vi "IdentificaçãoHost.vi"() -> ()   [LabVIEW 2018]
uses:
  Tanque.ctl
  SMHostEnum.ctl
  <vilib>/addons/System Identification/Model Typedefs.llb/si_generic model.ctl
  <vilib>/addons/System Identification/Model Typedefs.llb/SI Model Type.ctl
  <vilib>/addons/System Identification/Model Typedefs.llb/si_variables.ctl
  Setpoints.ctl
  PRBSparameters.ctl
  <vilib>/addons/System Identification/NI_SysID.lvlib
panel:
  in  "Amplitude":dbl=0.5
  in  "Update setpoints":bool
  out "Output 2":dbl[][](graph)
  out "Estimated MIMO State-space Model":picture
  out "Output 1":dbl[][](graph)
  in  "Excitation duration":i32=120
  in  "Period":i32=20
  in  "Pump seed 2":i32
  in  "Pump seed 1":i32
  in  "Coletar":bool
  out "Tanks levels variation":cluster{dbl, dbl, dbl, dbl}(graph)
  out "Pump voltage variation":cluster{dbl, dbl}(graph)
  in  "Valvula proporcional 2":dbl=7.5
  in  "Valvula proporcional 1":dbl=7.5
  out "Tanque 4":T1 scale=0.0..20.0
  out "Tanque 3":T1 scale=0.0..20.0
  out "Tanque 2":T1 scale=0.0..20.0
  out "Tanque 1":T1 scale=0.0..20.0
  in  "Valvula 4":bool
  in  "Valvula 3":bool
  in  "Valvula 1":bool
  in  "Valvula 2":bool
  in  "Pump 2":dbl=3.0 min=0.0 format="%.2f"
  in  "Pump 1":dbl=3.0 min=0.0 format="%.2f"
  # "Sistema Tanque Quádruplo"
  # "PRBS excitation signal"
  # "[0-10V]"
  # "[0-10V]"
  # "[0-10V]"
  # "[0-10V]"
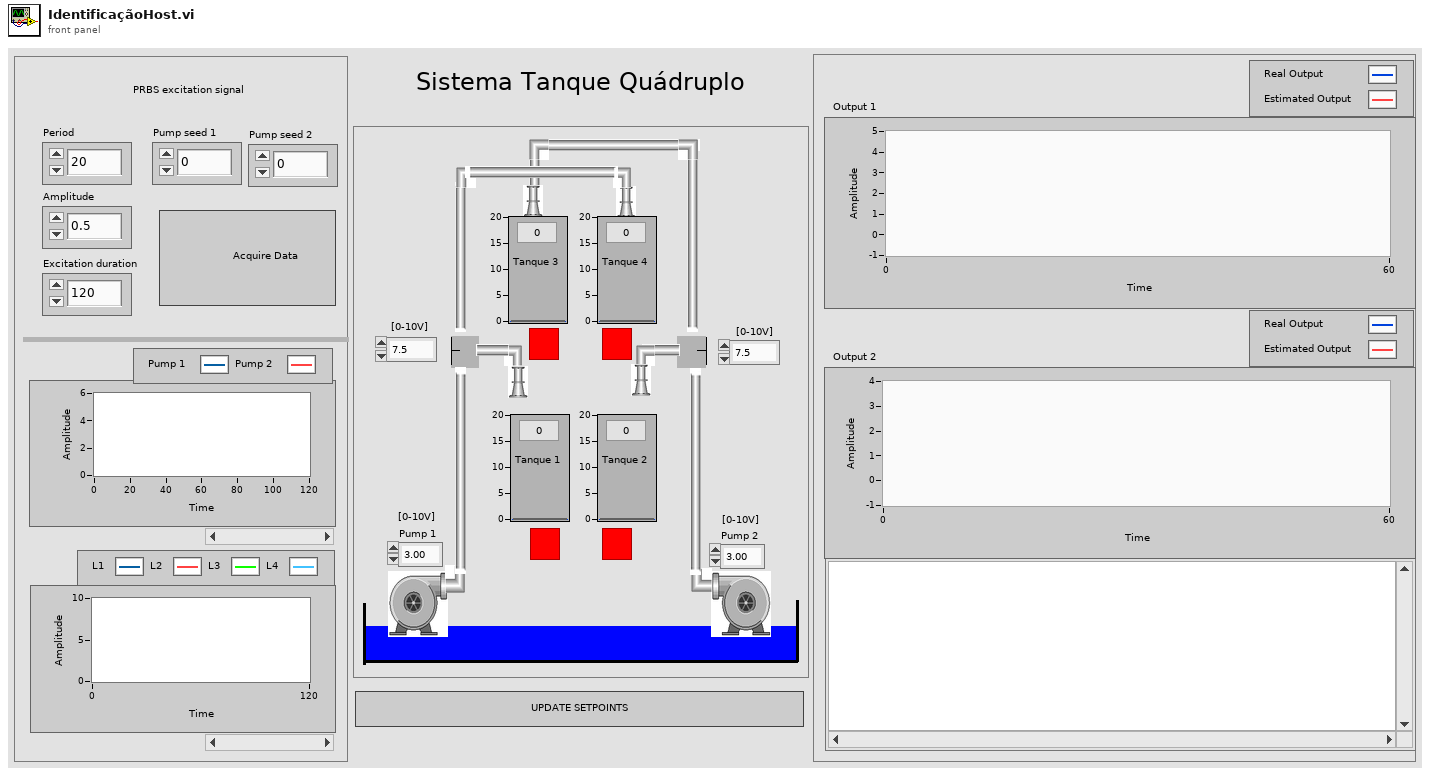
[diagram p1: front panel]
types:
  T1 = typedef "Tanque.ctl" = dbl
  T2 = typedef "SMHostEnum.ctl" = enum16{"Inicialização", "Pedir dados dos tanques", "Atualizar UI", "Configurar valores iniciais", "Começa aquisição", "Coletar dados", "Identificação", "Fecha arquivo log", "Data Logging", "Finalização"}
  T3 = typedef "Setpoints.ctl" = cluster{"Bomba 1":fxp<+/-,20,5>, "Bomba 2":fxp<+/-,20,5>, "Solenoide 1":bool, "Solenoide 2":bool, "Solenoide 3":bool, "Solenoide 4":bool, "Valvula proporcional 2":fxp<+/-,20,5>, "Valvula proporcional 1":fxp<+/-,20,5>}
  T4 = enum16{"open", "open or create", "create or replace", "create", "open (read-only)"}
  T5 = typedef "NI_SysID.lvlib/si_generic model.ctl" = cluster{"attributes":cluster{"version":string, "model type":T6, "input names":string[], "output names":string[], "notes":string}, "coefficients":cluster{"A ":dbl[][][], "B":dbl[][][], "F":dbl[][][], "C":dbl[][][], "D":dbl[][][]}, "std deviations":cluster{"A ":dbl[][][], "B":dbl[][][], "F":dbl[][][], "C":dbl[][][], "D":dbl[][][]}, "coefficients covariance":dbl[][][], "noise variance":dbl[][], "fs":dbl, "system info":cluster{"number of inputs":i32, "number of outputs":i32, "A order":i32[][], "B order":i32[][], "F order":i32[][], "C order":i32[][], "D order":i32[][], "Delays":i32[][]}, "kalman gain":dbl[][], "initial state":dbl[], "trans func":cluster{"betas":dbl[], "alphas":dbl[]}[][], "zeros-poles":cluster{"zeros":cdb[], "poles":cdb[], "gain":dbl}[][], "std of trans func":cluster{"betas":dbl[], "alphas":dbl[]}[][], "std of zeros-poles":cluster{"zeros":cdb[], "poles":cdb[], "gain":dbl}[][], "trans func (noise)":cluster{"betas":dbl[], "alphas":dbl[]}[][], "std of trans func (noise)":cluster{"betas":dbl[], "alphas":dbl[]}[][], "zeros-poles (noise)":cluster{"zeros":cdb[], "poles":cdb[], "gain":dbl}[][], "std of zeros-poles (noise)":cluster{"zeros":cdb[], "poles":cdb[], "gain":dbl}[][], "Symbolic State Space Model":cluster{"Symbolic A":string[][], "Symbolic B":string[][], "Symbolic C":string[][], "Symbolic D":string[][], "Symbolic K":string[][], "Symbolic Initial State":string[]}, "delay":dbl[][], "variables":T7, "grey trans func spec":cluster{"orders of TF model":cluster{" num order":i32, "den order":i32}, "# of zeros/poles at origin":cluster{"zeros/poles":u16, "number ":i32}, "delay initial?":bool, "gain initial?":bool}}
  T6 = typedef "NI_SysID.lvlib/SI Model Type.ctl" = u16
  T7 = typedef "NI_SysID.lvlib/si_variables.ctl" = cluster{"name":string, "initial guess":dbl, "upper limit":dbl, "lower limit":dbl, "value":dbl}[]
  T8 = enum8{"Enabled", "Disabled", "Disabled and Grayed Out"}
  T9 = typedef "PRBSparameters.ctl" = cluster{"seed":i64, "samples":i64, "upsampling factor":i32, "polynomial order":i32, "Amplitude":dbl}[]
  T10 = typedef "imagedata.ctl" = cluster{"image type":i32, "image depth":i32, "image":u8[], "mask":u8[], "colors":u32[], "Rectangle":cluster{"left":i16, "top":i16, "right":i16, "bottom":i16}}
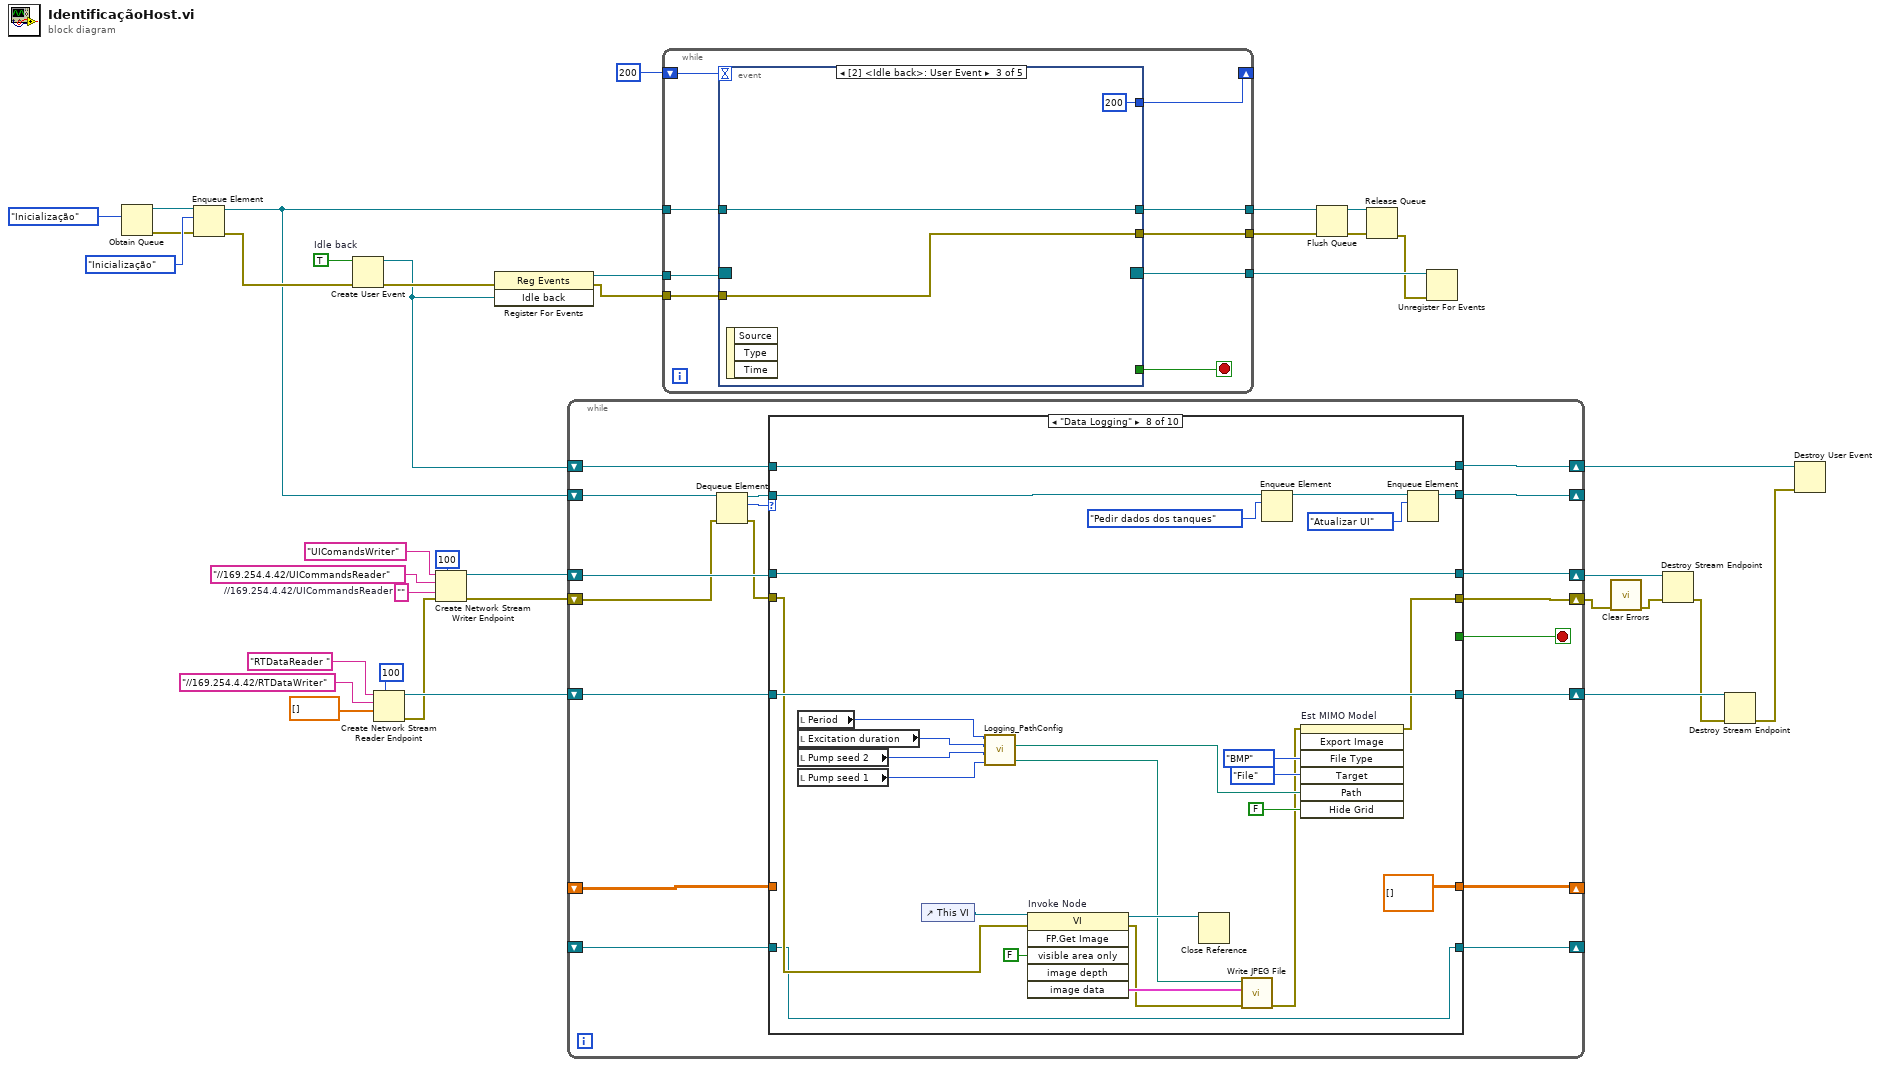
[diagram p0: block diagram]
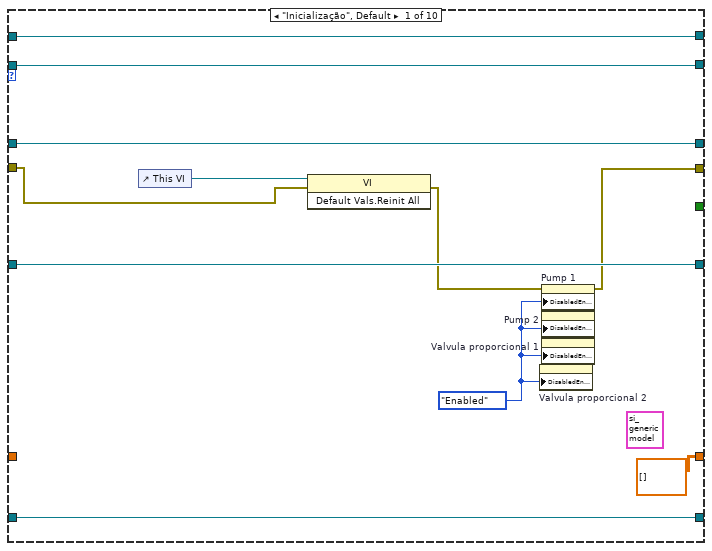
[diagram p2: hidden frame]
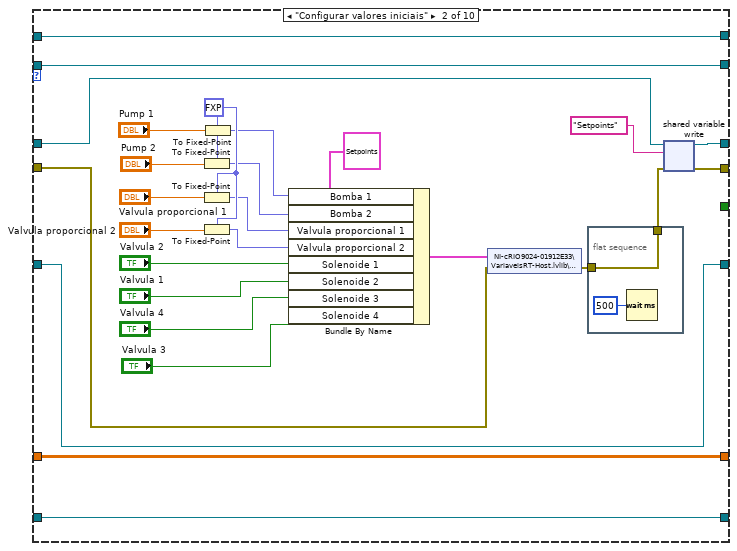
[diagram p3: hidden frame]
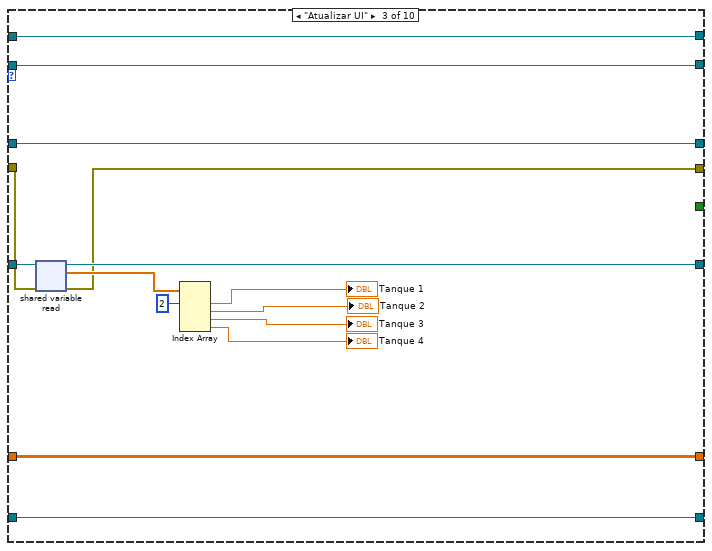
[diagram p4: hidden frame]
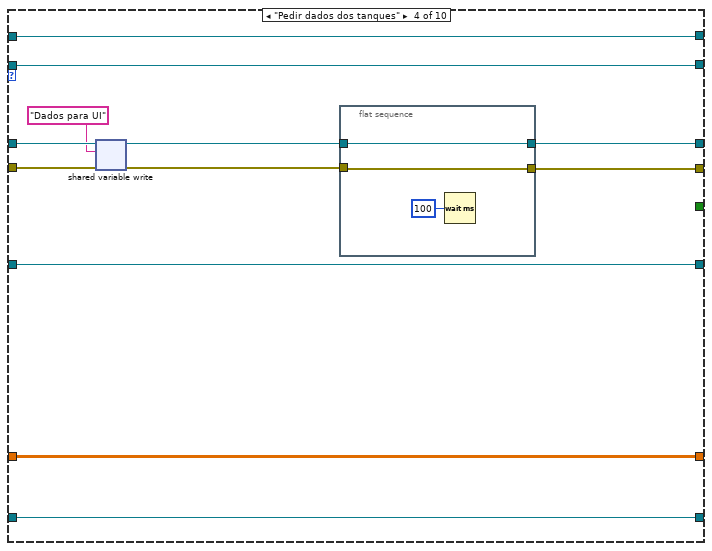
[diagram p5: hidden frame]
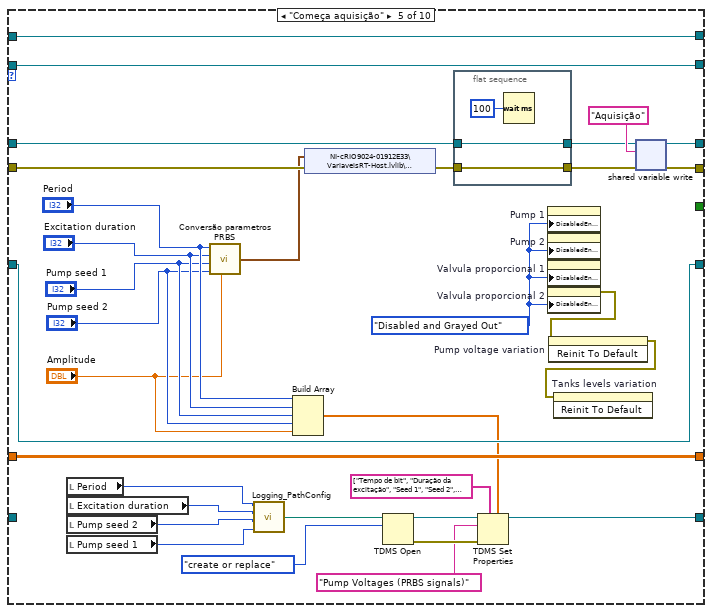
[diagram p6: hidden frame]
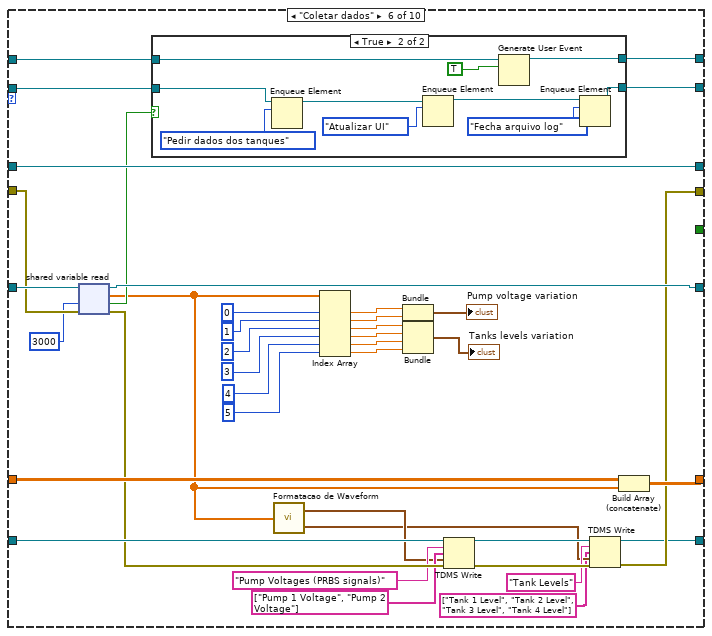
[diagram p7: hidden frame]
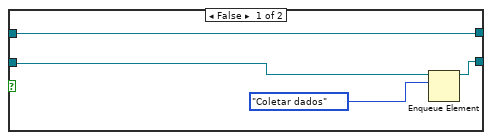
[diagram p8: hidden frame]
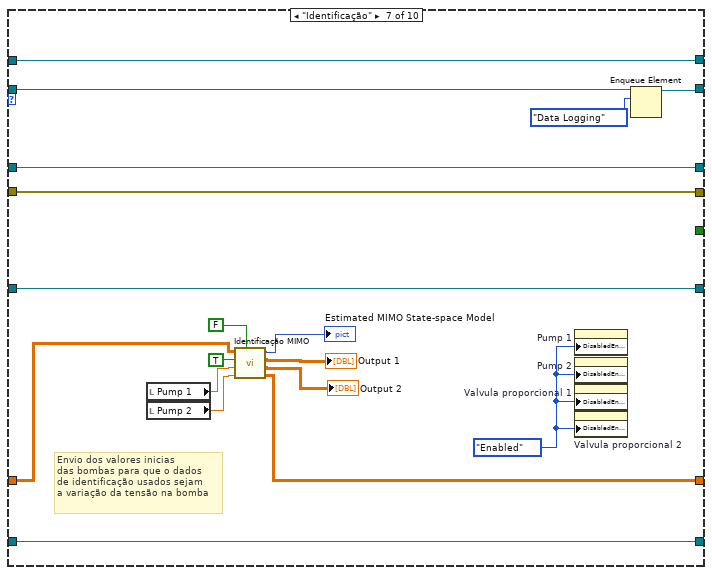
[diagram p9: hidden frame]
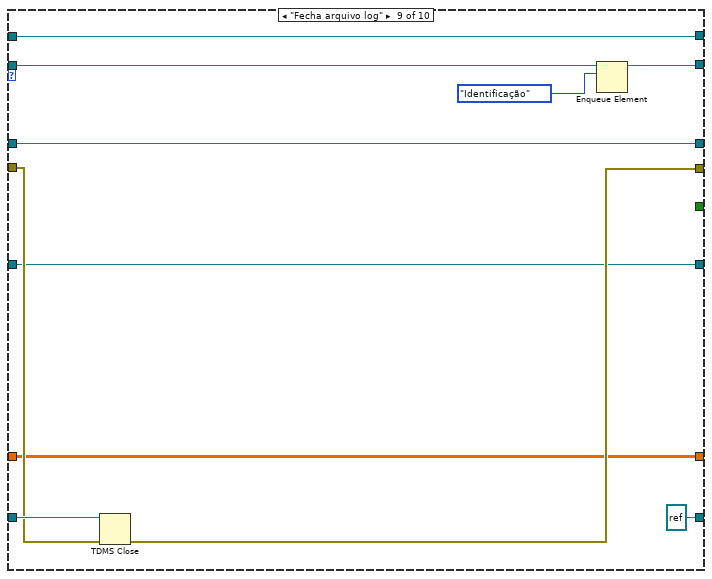
[diagram p10: hidden frame]
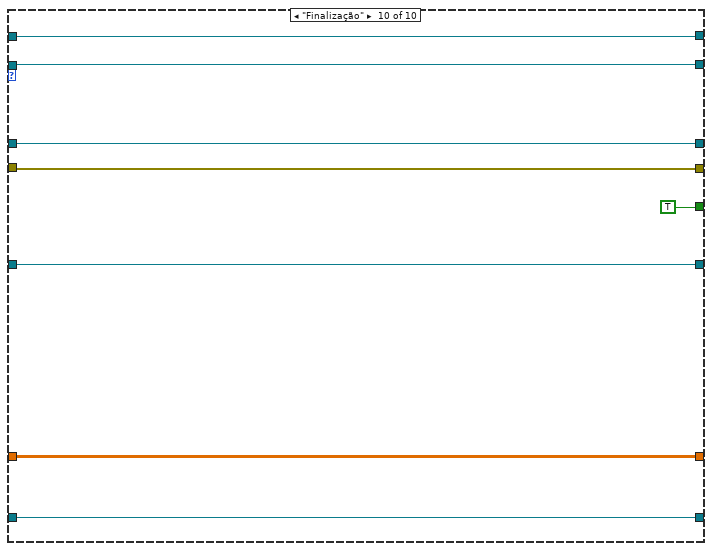
[diagram p11: hidden frame]
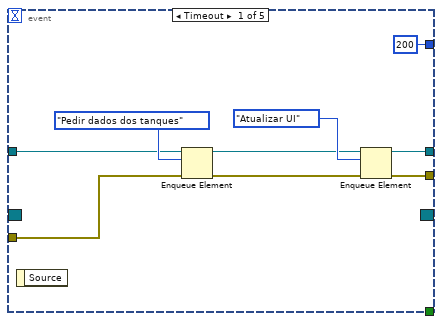
[diagram p12: hidden frame]
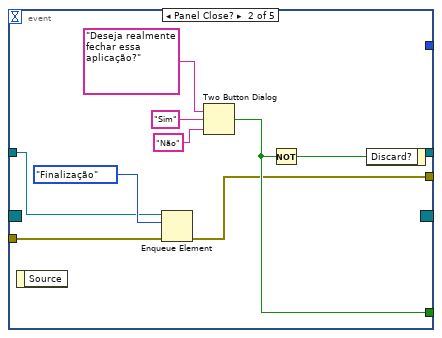
[diagram p13: hidden frame]
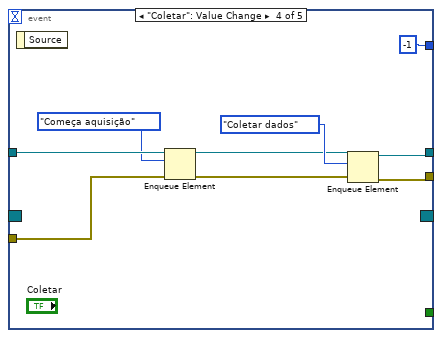
[diagram p14: hidden frame]
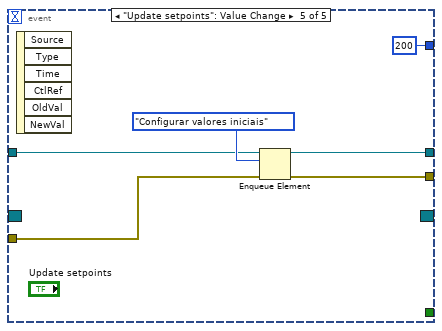
[diagram p15: hidden frame]
diagram:
  w19 = TRUE  # Idle back
  w26 = "//169.254.4.42/UICommandsReader"  # //169.254.4.42/UICommandsReader
  n1 = Obtain Queue(element data type=SMHostEnum."Inicialização") -> (queue out=w16:refnum<queue>, error out=w15:errorcluster)  [unwired: 4 in, 1 out]
  n2 = Enqueue Element(queue=w16, element=SMHostEnum."Inicialização", error in (no error)=w15) -> (queue out=w12:refnum<queue>, error out=w14:errorcluster)  [unwired: 1 in, 1 out]
  n3 = Create User Event(user event datatype=w19, error in=w14) -> (user event=w10:refnum<user-event>, error out=w17:errorcluster)
  n4 = Create Network Stream Reader Endpoint(7:100 ("reader buffer size"), 9:dbl[] [], 10:"//169.254.4.42/RTDataWriter" ("writer url"), 11:"RTDataReader " ("reader name")) -> (0:w23:errorcluster, 3:w33:refnum<k21>)  [unwired: 3 in]
  n5 = Create Network Stream Writer Endpoint(7:100 ("writer buffer size"), 8:w23, 9:"", 10:w26, 11:"UIComandsWriter") -> (0:w22:errorcluster, 3:w28:refnum<k21>)  [unwired: 2 in]
  n6 = register-events(error in=w17, w10) -> (reference out=w13:refnum<event-registration>, error out=w11:errorcluster)  [unwired: 1 in]
  n7 = while {
    shift-right: [w51] -> w6
    shift-left: w28 -> [w52]
    shift-right: [w39] -> w3
    shift-left: w22 -> [w45]
    shift-right: [w50] -> w5
    shift-left: w33 -> [w53]
    shift-right: [w48] -> _
    shift-left: w12 -> [w55]
    shift-right: [w47] -> _
    shift-left: _ -> [w46]
    shift-right: [w42] -> w7
    shift-left: w10 -> [w43]
    shift-right: [w41] -> _
    shift-left: _ -> [w40]
    stop <- w38 stop-if-true
    n8 = Dequeue Element(queue=w55, error in (no error)=w45) -> (queue out=w49:refnum<queue>, element=w54:T2, error out=w44:errorcluster)  [unwired: 1 in, 1 out]
    n9 = case shown="\"Data Logging\"" w54 {
      tunnel: w53 -> [w65 w75 w106 w119 w151 w200 w231 w255 w265 w275]
      tunnel: w44 -> [w60 w77 w100 w121 w157 w198 w230 w234 w269 w276]
      tunnel: w52 -> [w66 w80 w104 w122 w155 w199 w232 w254 w264 w277]
      tunnel: [w57 w78 w99 w115 w152 w169 w230 w235 w268 w276] -> w39
      tunnel: [w66 w76 w104 w116 w154 w199 w232 w254 w264 w277] -> w51
      tunnel: [w65 w75 w102 w119 w151 w194 w231 w255 w265 w275] -> w50
      tunnel: w49 -> [w64 w74 w101 w114 w150 w196 w227 w258 w261 w273]
      tunnel: [w64 w74 w101 w114 w150 w195 w228 w248 w260 w273] -> w48
      tunnel: [dbl[][] [] w71 w98 w113 w143 w179 w221 dbl[][] [] w266 w272] -> w47
      tunnel: w46 -> [_ w71 w98 w113 w143 w178 w216 _ w266 w272]
      tunnel: w43 -> [w62 w70 w97 w112 w149 w177 w226 w257 w263 w274]
      tunnel: [w62 w70 w97 w112 w149 w176 w226 w257 w263 w274] -> w42
      tunnel: [w56 w67 w96 w111 w127 w168 w215 w233 refnum<k34> refnum ("tdms file out") w271] -> w41
      tunnel: w40 -> [w56 w67 w96 w111 _ w174 w215 w233 w270 w271]
      tunnel: [_ _ _ _ _ _ _ _ _ TRUE] -> w38
      frame "Inicialização", Default {
        (unwired) T5 {"attributes"={"version"="v3.0", "model type"=0, "input names"=[], "output names"=[], "notes"=""}, "coefficients"={"A "=[], "B"=[], "F"=[], "C"=[], "D"=[]}, "std deviations"={"A "=[], "B"=[], "F"=[], "C"=[], "D"=[]}, "coefficients covariance"=[], "noise variance"=[], "fs"=0.0, "system info"={"number of inputs"=0, "number of outputs"=0, "A order"=[], "B order"=[], "F order"=[], "C order"=[], "D order"=[], "Delays"=[]}, "kalman gain"=[], "initial state"=[], "trans func"=[], "zeros-poles"=[], "std of trans func"=[], "std of zeros-poles"=[], "trans func (noise)"=[], "std of trans func (noise)"=[], "zeros-poles (noise)"=[], "std of zeros-poles (noise)"=[], "Symbolic State Space Model"={"Symbolic A"=[], "Symbolic B"=[], "Symbolic C"=[], "Symbolic D"=[], "Symbolic K"=[], "Symbolic Initial State"=[]}, "delay"=[], "variables"=[], "grey trans func spec"={"orders of TF model"={" num order"=1, "den order"=2}, "# of zeros/poles at origin"={"zeros/poles"=1, "number "=0}, "delay initial?"=FALSE, "gain initial?"=FALSE}} ("system model out")
        w59 = T8."Enabled" ("Disabled")
        n10 = control-ref of="This VI"() -> (w61:refnum<vi>)
        n11 = invoke class="VI" method="Default Vals.Reinit All"(reference=w61, error in=w60) -> (error out=w58:errorcluster)  [unwired: 1 in, 2 out]
        n12 = property on="Valvula proporcional 2" class="DigNum (strict)"("DisabledEnum"=w59) -> ()  [unwired: 2 in, 2 out]
        n13 = property on="Pump 1" class="DigNum (strict)"(error in=w58, "DisabledEnum"=w59) -> (error out=w57:errorcluster)  [unwired: 1 in, 1 out]
        n14 = property on="Pump 2" class="DigNum (strict)"("DisabledEnum"=w59) -> ()  [unwired: 2 in, 2 out]
        n15 = property on="Valvula proporcional 1" class="DigNum (strict)"("DisabledEnum"=w59) -> ()  [unwired: 2 in, 2 out]
      }
      frame "Configurar valores iniciais" {
        w91 = fxp<+/-,20,5> 0.0 ("fixed-point type")
        n16 = To Fixed-Point(fixed-point type=w91, number="Pump 2") -> (fixed-point=w88:fxp<+/-,20,5>)
        n17 = To Fixed-Point(fixed-point type=w91, number="Valvula proporcional 1") -> (fixed-point=w89:fxp<+/-,20,5>)
        n18 = To Fixed-Point(fixed-point type=w91, number="Valvula proporcional 2") -> (fixed-point=w90:fxp<+/-,20,5>)
        n19 = To Fixed-Point(fixed-point type=w91, number="Pump 1") -> (fixed-point=w87:fxp<+/-,20,5>)
        n20 = Bundle By Name(cluster=T3 {"Bomba 1"=0.0, "Bomba 2"=0.0, "Solenoide 1"=FALSE, "Solenoide 2"=FALSE, "Solenoide 3"=FALSE, "Solenoide 4"=FALSE, "Valvula proporcional 2"=0.0, "Valvula proporcional 1"=0.0} ("Cluster"), "Bomba 1"=w87, "Bomba 2"=w88, "Valvula proporcional 1"=w89, "Valvula proporcional 2"=w90, "Solenoide 1"="Valvula 2", "Solenoide 2"="Valvula 1", "Solenoide 3"="Valvula 4", "Solenoide 4"="Valvula 3") -> (w93:T3)
        n21 = shared-variable "NI-cRIO9024-01912E33\\VariaveisRT-Host.lvlib\\Setpoints"(w93, error in=w77) -> (error out=w73:errorcluster)
        n22 = flat-sequence {
          tunnel: w73 -> [w94]
          tunnel: [w94] -> w72
          frame #0 {
            n23 = Wait (ms)(milliseconds to wait=u32 500) -> ()  [unwired: 1 out]
          }
        }
        n24 = shared-variable-write(w80, w72, "Setpoints" ("data in")) -> (w76:refnum<k21>, w78:errorcluster)  [unwired: 1 in, 1 out]
      }
      frame "Atualizar UI" {
        n25 = shared-variable-read(w106, w100) -> (w102:refnum<k21>, w99:errorcluster, w103:dbl[])  [unwired: 1 in, 1 out]
        n26 = Index Array(array=w103, index #1=2 ("index")) -> (element #1=→"Tanque 1":dbl, element #2=→"Tanque 2":dbl, element #3=→"Tanque 3":dbl, element #4=→"Tanque 4":dbl)  [unwired: 3 in]
      }
      frame "Pedir dados dos tanques" {
        n27 = shared-variable-write(w122, w121, "Dados para UI" ("data in")) -> (w118:refnum<k21>, w117:errorcluster)  [unwired: 1 in, 1 out]
        n28 = flat-sequence {
          tunnel: w118 -> [w125]
          tunnel: w117 -> [w124]
          tunnel: [w125] -> w116
          tunnel: [w124] -> w115
          frame #0 {
            n29 = Wait (ms)(milliseconds to wait=u32 100) -> ()  [unwired: 1 out]
          }
        }
      }
      frame "Começa aquisição" {
        w148 = T8."Disabled and Grayed Out" ("Disabled")
        n30 = local read "Period"() -> (w142:i32)
        n31 = local read "Excitation duration"() -> (w141:i32)
        n32 = local read "Pump seed 2"() -> (w140:i32)
        n33 = local read "Pump seed 1"() -> (w139:i32)
        n34 = call "Conversão parametros PRBS.vi"("Amplitude"="Amplitude", "Seed bomba 2"="Pump seed 2", "Seed bomba 1"="Pump seed 1", "Duração da excitação (s)"="Excitation duration", "Periodo"="Period") -> ("PRBS Parameters 2"=w144:T9)  [unwired: 1 in]
        n35 = call "Logging_PathConfig.vi"("Period"=w142, "Excitation Duration"=w141, "Seed1"=w140, "Seed2"=w139) -> ("Data path 2"=w138:path)  [unwired: 1 in, 2 out]
        n36 = Build Array("Period", "Excitation duration", "Pump seed 1", "Pump seed 2", "Amplitude") -> (w130:dbl[])
        n37 = shared-variable "NI-cRIO9024-01912E33\\VariaveisRT-Host.lvlib\\PRBSparameters"(w144, error in=w157) -> (error out=w147:errorcluster)
        n38 = TDMS Open(10:T4."create or replace" ("operation (0:open)"), 11:w138) -> (0:w128:errorcluster, 3:w129:refnum<k34>)  [unwired: 5 in]
        n39 = flat-sequence {
          tunnel: w147 -> [w159]
          tunnel: [w160] -> w156
          tunnel: w155 -> [w160]
          tunnel: [w159] -> w153
          frame #0 {
            n40 = Wait (ms)(milliseconds to wait=u32 100) -> ()  [unwired: 1 out]
          }
        }
        n41 = TDMS Set Properties(5:w130, 7:string[] ["Tempo de bit", "Duração da excitação", "Seed 1", "Seed 2", "Amplitude"] ("property names"), 8:w128, 10:"Pump Voltages (PRBS signals)" ("group name"), 11:w129) -> (3:w127:refnum<k34>)  [unwired: 1 in, 3 out]
        n42 = property on="Pump 1" class="DigNum (strict)"("DisabledEnum"=w148) -> ()  [unwired: 2 in, 2 out]
        n43 = property on="Pump 2" class="DigNum (strict)"("DisabledEnum"=w148) -> ()  [unwired: 2 in, 2 out]
        n44 = property on="Valvula proporcional 1" class="DigNum (strict)"("DisabledEnum"=w148) -> ()  [unwired: 2 in, 2 out]
        n45 = property on="Valvula proporcional 2" class="DigNum (strict)"("DisabledEnum"=w148) -> (error out=w146:errorcluster)  [unwired: 2 in, 1 out]
        n46 = invoke on="Pump voltage variation" class="WFChart (strict)" method="Reinit To Default"(error in=w146) -> (error out=w145:errorcluster)  [unwired: 2 in, 2 out]
        n47 = invoke on="Tanks levels variation" class="WFChart (strict)" method="Reinit To Default"(error in=w145) -> ()  [unwired: 2 in, 3 out]
        n48 = shared-variable-write(w156, w153, "Aquisição" ("data in")) -> (w154:refnum<k21>, w152:errorcluster)  [unwired: 1 in, 1 out]
      }
      frame "Coletar dados" {
        n49 = shared-variable-read(w200, w198, 3000 ("timeout ms (-1)")) -> (w194:refnum<k21>, w173:errorcluster, w175:bool, w163:dbl[])
        n50 = case shown="True" w175 {
          tunnel: w196 -> [w203 w206]
          tunnel: [w202 w209] -> w195
          tunnel: w177 -> [w201 w213]
          tunnel: [w201 w211] -> w176
          frame False {
            n51 = Enqueue Element(queue=w203, element=SMHostEnum."Coletar dados") -> (queue out=w202:refnum<queue>)  [unwired: 2 in, 2 out]
          }
          frame True {
            n52 = Enqueue Element(queue=w206, element=SMHostEnum."Pedir dados dos tanques") -> (queue out=w207:refnum<queue>)  [unwired: 2 in, 2 out]
            n53 = Enqueue Element(queue=w207, element=SMHostEnum."Atualizar UI") -> (queue out=w210:refnum<queue>)  [unwired: 2 in, 2 out]
            n54 = Generate User Event(user event=w213, event data cluster=TRUE ("event data")) -> (user event out=w211:refnum<user-event>)  [unwired: 2 in, 1 out]
            n55 = Enqueue Element(queue=w210, element=SMHostEnum."Fecha arquivo log") -> (queue out=w209:refnum<queue>)  [unwired: 2 in, 2 out]
          }
        }
        n56 = call "Formatacao de Waveform.vi"("Array in"=w163) -> ("Tank Levels"=w164:waveform(dbl)[], "Pump Voltages"=w165:waveform(dbl)[])  [unwired: 2 in]
        n57 = Index Array(array=w163, index #1=0 ("index (row)"), index #2=1 ("index (row)"), index #3=2 ("index (row)"), index #4=3 ("index (row)"), index #5=4 ("index (row)"), index #6=5 ("index (row)")) -> (element #1=w187:dbl, element #2=w186:dbl, element #3=w185:dbl, element #4=w184:dbl, element #5=w182:dbl, element #6=w183:dbl)
        n58 = Bundle(w187, w186) -> (→"Pump voltage variation":cluster{dbl, dbl})  [unwired: 1 in]
        n59 = Bundle(w185, w184, w182, w183) -> (→"Tanks levels variation":cluster{dbl, dbl, dbl, dbl})  [unwired: 1 in]
        n60 = TDMS Write(0:w174, 5:"Pump Voltages (PRBS signals)" ("group name in (Untitled)"), 7:string[] ["Pump 1 Voltage", "Pump 2 Voltage"], 9:w165, 11:w173) -> (4:w171:refnum<k34>, 15:w170:errorcluster)  [unwired: 1 in, 2 out]
        n61 = TDMS Write(0:w171, 5:"Tank Levels" ("group name in (Untitled)"), 7:string[] ["Tank 1 Level", "Tank 2 Level", "Tank 3 Level", "Tank 4 Level"], 9:w164, 11:w170) -> (4:w168:refnum<k34>, 15:w169:errorcluster)  [unwired: 1 in, 2 out]
        n62 = Build Array (concatenate)(w178, w163) -> (w179:dbl[][])
      }
      frame "Identificação" {
        w225 = T8."Enabled" ("Disabled")
        # "Envio dos valores inicias\ndas bombas para que o dados \nde identificação usados sejam \na variação da tensão na bomba"
        n63 = local read "Pump 1"() -> (w219:dbl)
        n64 = local read "Pump 2"() -> (w220:dbl)
        n65 = call "Identificação MIMO.vi"("Remove Trend"=FALSE, "Init Pump 2 voltage"=w220, "Init Pump 1 voltage"=w219, "Invert indentification and validation data?"=TRUE, "Stimulus and Response Signal"=w216) -> ("Acquired and identification signals"=w221:dbl[][], "output 2"=→"Output 2":dbl[][], "output 1"=→"Output 1":dbl[][], "Estimated MIMO State-space Model"=→"Estimated MIMO State-space Model":picture)  [unwired: 2 in, 1 out]
        n66 = property on="Pump 1" class="DigNum (strict)"("DisabledEnum"=w225) -> ()  [unwired: 2 in, 2 out]
        n67 = property on="Pump 2" class="DigNum (strict)"("DisabledEnum"=w225) -> ()  [unwired: 2 in, 2 out]
        n68 = property on="Valvula proporcional 1" class="DigNum (strict)"("DisabledEnum"=w225) -> ()  [unwired: 2 in, 2 out]
        n69 = property on="Valvula proporcional 2" class="DigNum (strict)"("DisabledEnum"=w225) -> ()  [unwired: 2 in, 2 out]
        n70 = Enqueue Element(queue=w227, element=SMHostEnum."Data Logging") -> (queue out=w228:refnum<queue>)  [unwired: 2 in, 2 out]
      }
      frame "Data Logging" {
        n71 = local read "Period"() -> (w244:i32)
        n72 = local read "Excitation duration"() -> (w243:i32)
        n73 = local read "Pump seed 2"() -> (w242:i32)
        n74 = local read "Pump seed 1"() -> (w241:i32)
        n75 = control-ref of="This VI"() -> (w247:refnum<vi>)
        n76 = call "Logging_PathConfig.vi"("Period"=w244, "Excitation Duration"=w243, "Seed1"=w242, "Seed2"=w241) -> ("Model path"=w240:path, "Front panel image path"=w237:path)  [unwired: 1 in, 1 out]
        n77 = invoke on="Invoke Node" class="VI" method="FP.Get Image"(reference=w247, error in=w234, "visible area only"=FALSE ("Visible Area Only")) -> (reference out=w246:refnum<vi>, error out=w236:errorcluster, "image data"=w245:T10)  [unwired: 3 in, 3 out]
        n78 = Close Reference(reference=w246) -> ()  [unwired: 1 in, 1 out]
        n79 = call <vilib>:"Write JPEG File.vi"("error in (no error)"=w236, "image data"=w245, "path to JPEG file"=w237) -> ("error out"=w238:errorcluster)  [unwired: 7 in, 1 out]
        n80 = Enqueue Element(queue=w258, element=SMHostEnum."Pedir dados dos tanques") -> (queue out=w249:refnum<queue>)  [unwired: 2 in, 2 out]
        n81 = invoke on="Est MIMO Model" class="Pict" method="Export Image"(error in=w238, "File Type"=enum32{"BMP", "EPS", "EMF", "PICT"}."BMP", "Target"=enum32{"File", "Clipboard"}."File", "Path"=w240, "Hide Grid"=FALSE ("Always Overwrite")) -> (error out=w235:errorcluster)  [unwired: 2 in, 6 out]
        n82 = Enqueue Element(queue=w249, element=SMHostEnum."Atualizar UI") -> (queue out=w248:refnum<queue>)  [unwired: 2 in, 2 out]
      }
      frame "Fecha arquivo log" {
        n83 = TDMS Close(8:w269, 11:w270) -> (0:w268:errorcluster)  [unwired: 1 out]
        n84 = Enqueue Element(queue=w261, element=SMHostEnum."Identificação") -> (queue out=w260:refnum<queue>)  [unwired: 2 in, 2 out]
      }
      frame "Finalização" {
      }
    }
  }
  n85 = while {
    tunnel: w12 -> [w287]
    tunnel: [w286] -> w35
    tunnel: [w285] -> w34
    shift-right: [w283] -> _
    shift-left: 200 -> [w284]
    tunnel: w13 -> [w281]
    tunnel: w11 -> [w280]
    tunnel: [w279] -> w9
    stop <- w282 stop-if-true
    n86 = event shown="[2] <Idle back>: User Event" {
      selector: w281 -> [_ _ _ _ _]
      dyn-events: [_ _ _ _ _] -> w279
      timeout: w284 -> [_ _ _ _ _]
      tunnel: w287 -> [w295 w297 w308 w317 w322]
      tunnel: w280 -> [w294 w299 w307 w309 w321]
      tunnel: [w290 _ w308 w312 w320] -> w286
      tunnel: [w289 w298 w307 w310 w319] -> w285
      tunnel: [200 _ 200 -1 200] -> w283
      tunnel: [_ w301 _ _ _] -> w282
      event Timeout {
        n87 = event-data() -> ()  [unwired: 1 in, 1 out]
        n88 = Enqueue Element(queue=w295, element=SMHostEnum."Pedir dados dos tanques", error in (no error)=w294) -> (queue out=w291:refnum<queue>, error out=w288:errorcluster)  [unwired: 1 in, 1 out]
        n89 = Enqueue Element(queue=w291, element=SMHostEnum."Atualizar UI", error in (no error)=w288) -> (queue out=w290:refnum<queue>, error out=w289:errorcluster)  [unwired: 1 in, 1 out]
      }
      event Panel Close? {
        n90 = event-data() -> ()  [unwired: 1 in, 1 out]
        n91 = Enqueue Element(queue=w297, element=SMHostEnum."Finalização", error in (no error)=w299) -> (error out=w298:errorcluster)  [unwired: 1 in, 2 out]
        n92 = Two Button Dialog(message="Deseja realmente fechar essa aplicação?", 1:"Não" ("F button name (\"Cancel\")"), 2:"Sim" ("T button name (\"OK\")")) -> (T button?=w301:bool)
        n93 = Not(x=w301) -> (.not. x?=w302:bool)
        n94 = event-data("Discard?"=w302) -> ()  [unwired: 1 in, 1 out]
      }
      event User Event {
        n95 = event-data() -> ()  [unwired: 1 in, 3 out]
      }
      event "Coletar": Value Change {
        n96 = event-data() -> ()  [unwired: 1 in, 1 out]
        n97 = Enqueue Element(queue=w317, element=SMHostEnum."Começa aquisição", error in (no error)=w309) -> (queue out=w313:refnum<queue>, error out=w311:errorcluster)  [unwired: 1 in, 1 out]
        n98 = Enqueue Element(queue=w313, element=SMHostEnum."Coletar dados", error in (no error)=w311) -> (queue out=w312:refnum<queue>, error out=w310:errorcluster)  [unwired: 1 in, 1 out]
      }
      event "Update setpoints": Value Change {
        n99 = event-data() -> ()  [unwired: 1 in, 6 out]
        n100 = Enqueue Element(queue=w322, element=SMHostEnum."Configurar valores iniciais", error in (no error)=w321) -> (queue out=w320:refnum<queue>, error out=w319:errorcluster)  [unwired: 1 in, 1 out]
      }
    }
  }
  n101 = Flush Queue(queue=w35, error in (no error)=w34) -> (queue out=w37:refnum<queue>, error out=w36:errorcluster)  [unwired: 1 out]
  n102 = Release Queue(queue=w37, error in (no error)=w36) -> (error out=w8:errorcluster)  [unwired: 1 in, 2 out]
  n103 = Unregister For Events(event registration refnum=w9, error in=w8) -> ()  [unwired: 1 out]
  n104 = call <vilib>:"Clear Errors.vi"("error in (no error)"=w3) -> ("error out"=w4:errorcluster)  [unwired: 5 in, 1 out]
  n105 = Destroy Stream Endpoint(8:w4, 11:w6) -> (0:w2:errorcluster)
  n106 = Destroy Stream Endpoint(8:w2, 11:w5) -> (0:w1:errorcluster)
  n107 = Destroy User Event(user event=w7, error in=w1) -> ()  [unwired: 1 out]
